vi "Panel.vi"(11 "ButtonControlEditorPanel in":refnum<class "ButtonControlEditorPanel.lvclass">) -> ()   [LabVIEW 2020, in "VolatusGUIControls.lvlib" / "ButtonControlEditorPanel.lvclass"]
uses:
  ButtonControlEditorPanel.lvclass
  C:/dev/lv20CE/relink/volatus-gui-controls/VolatusGUIEditorCore/ElementEditorPanel/ElementEditorPanel.lvclass
  C:/dev/lv20CE/relink/lv-oopanel/OOPanel/Panel/Panel.lvclass
  lv-oopanel/OOPanel/Panel/Basic UI State.ctl
  lv-autocomplete/AutoComplete/AutoComplete/AutoComplete.lvclass/AutoComplete.ctl
  ButtonControlEditorPanel.lvclass/ButtonControlEditorPanel.ctl
  31a50c44-4b6b-485d-bc13-bfcd23764fd1.vi
  03e8aef8-299f-4e90-a8ff-d58387ca9363.vi
  lv-autocomplete/AutoComplete/Launch Autocomplete Handler.vi
  <vilib>/JDP Science/JSONtext/Variant to JSON Text.vi
  <vilib>/JDP Science/JSONtext/Set Item.vi
  <vilib>/JDP Science/JSONtext/Pretty Print.vi
  lv-autocomplete/AutoComplete/AutoComplete/AutoComplete.lvclass
  <vilib>/JDP Science/JSONtext/LVClass Serializer/JSONtext LVClass Serializer.lvclass
  lv-oopanel/OOPanel/Panel/Panel.lvclass
  lv-oopanel/OOPanel/OOPanel.lvlib
  VolatusGUIControls.lvlib
  VolatusGUIEditorCore/ElementEditorPanel/ElementEditorPanel.lvclass
  VolatusGUIEditorCore/VolatusGUIEditorCore.lvlib
panel:
  in  "Inhibit":string caption="Channel"
  in  "Top":i32
  in  "Left":i32
  in  "Height":u16
  in  "Width":u16
  in  "Label Text Color":u32(colorbox) caption="Color"
  in  "Text Color":u32(colorbox)
  in  "Label Visible":bool caption="Visible"
  in  "Label":string
  in  "Multi":bool
  in  "Channel":string
  in  "True Color":u32(colorbox)
  in  "False Color":u32(colorbox)
  in  "True Text":string
  in  "False Text":string
  # "Label"
  # "False"
  # "True"
  # "Text"
  # "BG"
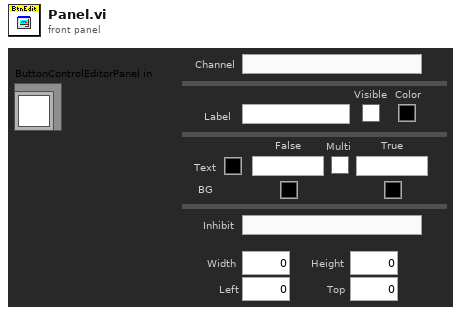
[diagram p1: front panel]
types:
  T1 = typedef "OOPanel.lvlib/Panel.lvclass/Basic UI State.ctl" = enum16{"Init", "Run", "Close"}
  T2 = typedef "VolatusGUIEditorCore.lvlib/ElementEditorPanel.lvclass/Incoming Events.ctl" = cluster{"Update Control":refnum<user-event>}
  T3 = typedef "OOPanel.lvlib/Panel.lvclass/Panel Events.ctl" = cluster{"Visbility":refnum<user-event>, "Close":refnum<user-event>}
  T4 = typedef "VolatusGUIControls.lvlib/ButtonControlEditorPanel.lvclass/Props.ctl" = cluster{"JSON":T5, "Label":T6, "Position":T7, "Width":u16, "Height":u16, "Boolean Colors":T8, "Boolean Text Props":T9}
  T5 = typedef "VolatusGUIControls.lvlib/ButtonControlEditorPanel.lvclass/JSON Props.ctl" = cluster{"Channel":string, "Inhibit":string}
  T6 = typedef "VolatusGUIEditorCore.lvlib/Label Props.ctl" = cluster{"Text":string, "Text Color":u32, "Visible":bool}
  T7 = typedef "VolatusGUIEditorCore.lvlib/Position Props.ctl" = cluster{"Left":i32, "Top":i32}
  T8 = typedef "VolatusGUIEditorCore.lvlib/Boolean Color Props.ctl" = cluster{"False":u32, "True":u32}
  T9 = typedef "VolatusGUIEditorCore.lvlib/Boolean Text Props.ctl" = cluster{"Color":u32, "MultiString":bool, "False":string, "True":string, "Visible":bool}
  T10 = typedef "OOPanel.lvlib/Visibility State.ctl" = enum16{"Idle", "Closed", "Hidden", "Visible", "Subpanel", "Hidden Subpanel"}
  T11 = cluster{"Label":string, "Label Text Color":u32, "Label Visible":bool}
  T12 = cluster{"Text Color":u32, "Multi":bool, "False Text":string, "True Text":string, "Visible":bool}
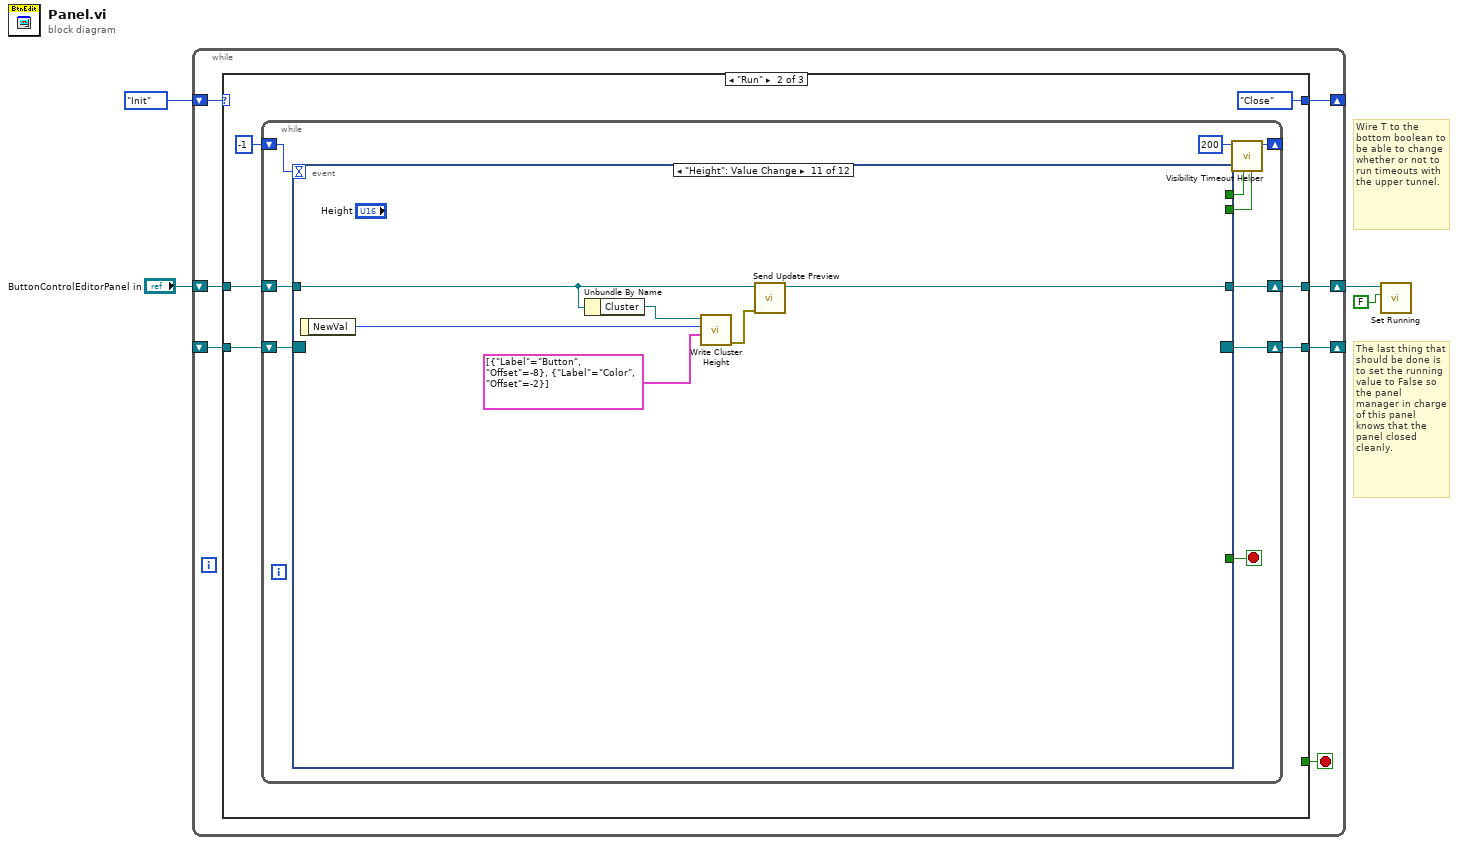
[diagram p0: block diagram]
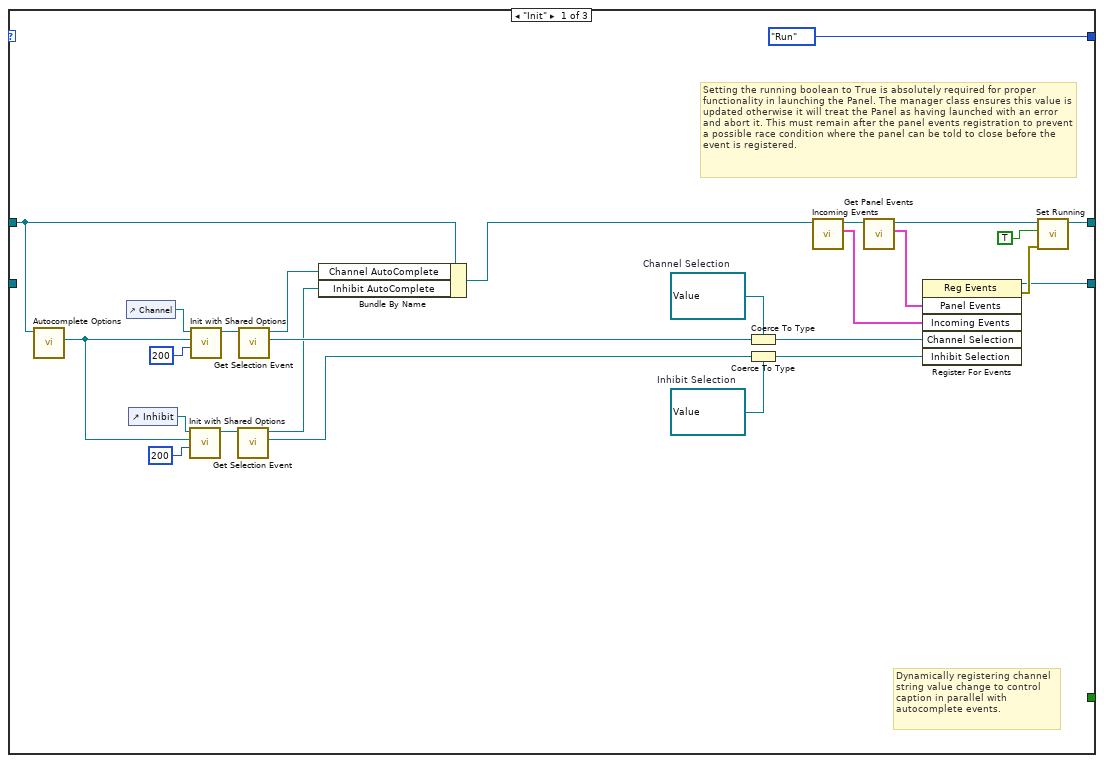
[diagram p2: hidden frame]
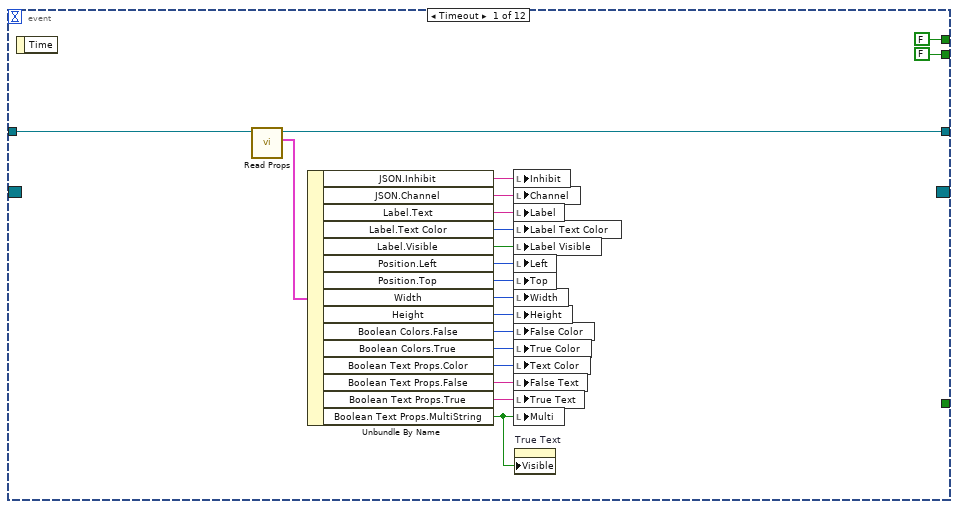
[diagram p3: hidden frame]
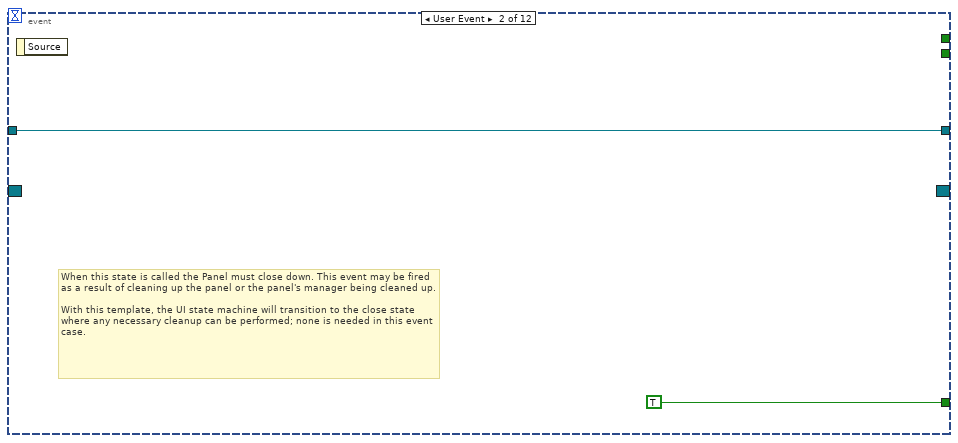
[diagram p4: hidden frame]
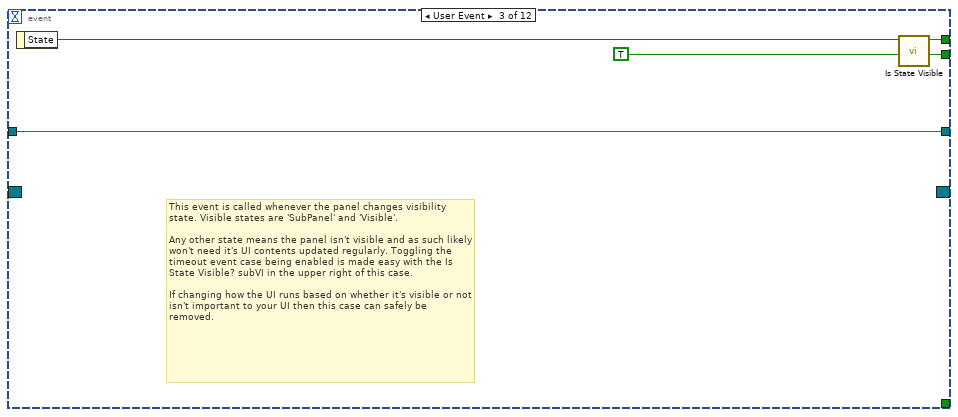
[diagram p5: hidden frame]
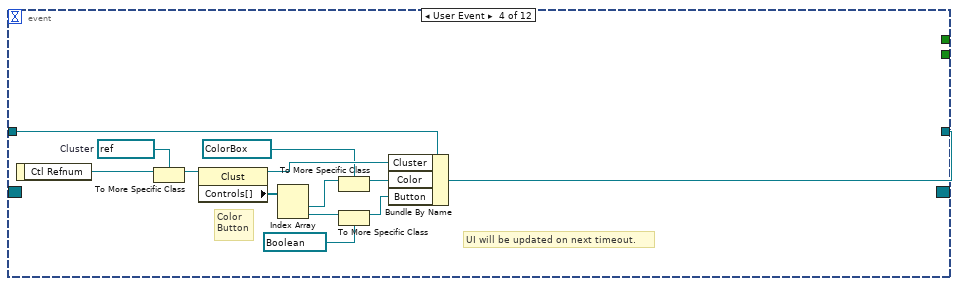
[diagram p6: hidden frame]
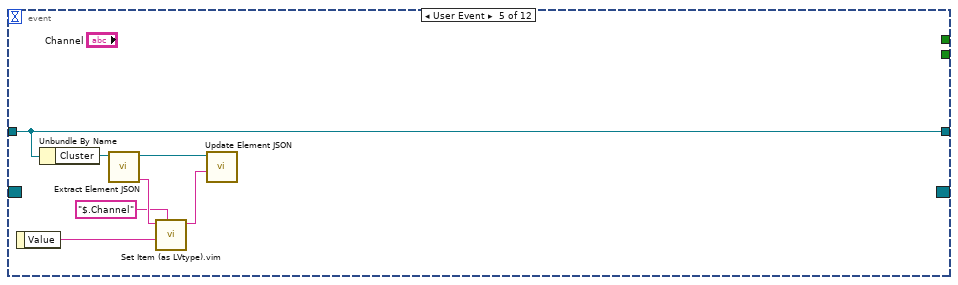
[diagram p7: hidden frame]
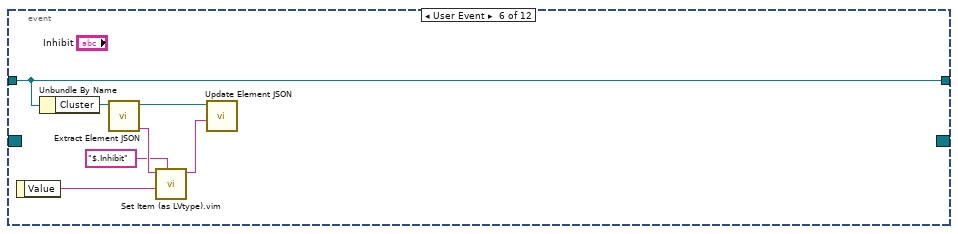
[diagram p8: hidden frame]
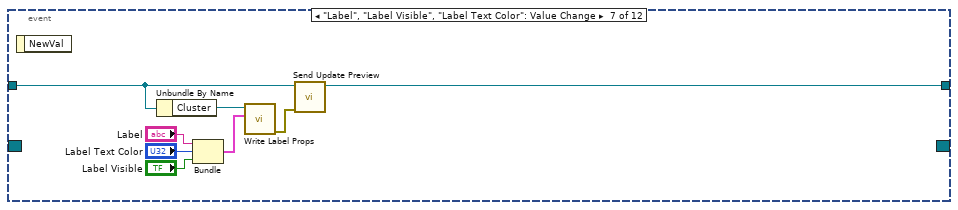
[diagram p9: hidden frame]
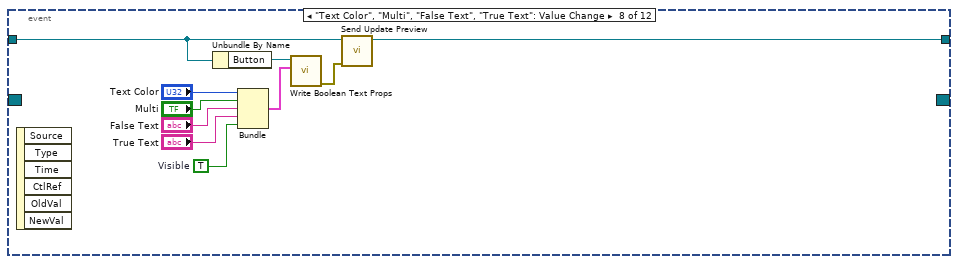
[diagram p10: hidden frame]
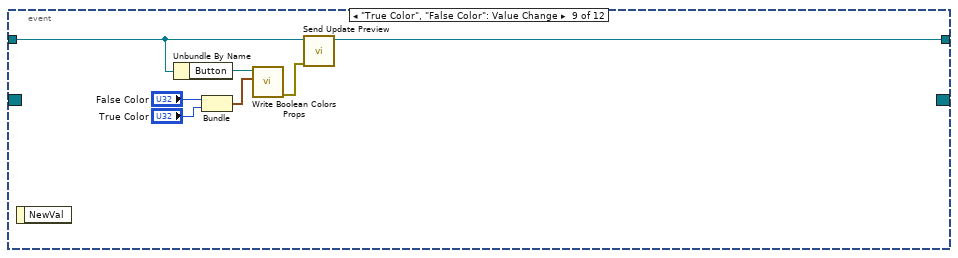
[diagram p11: hidden frame]
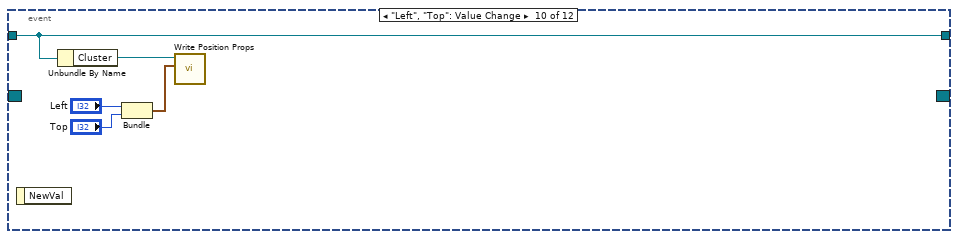
[diagram p12: hidden frame]
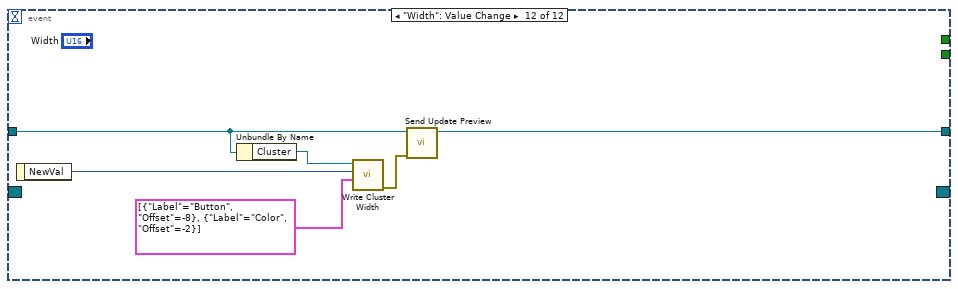
[diagram p13: hidden frame]
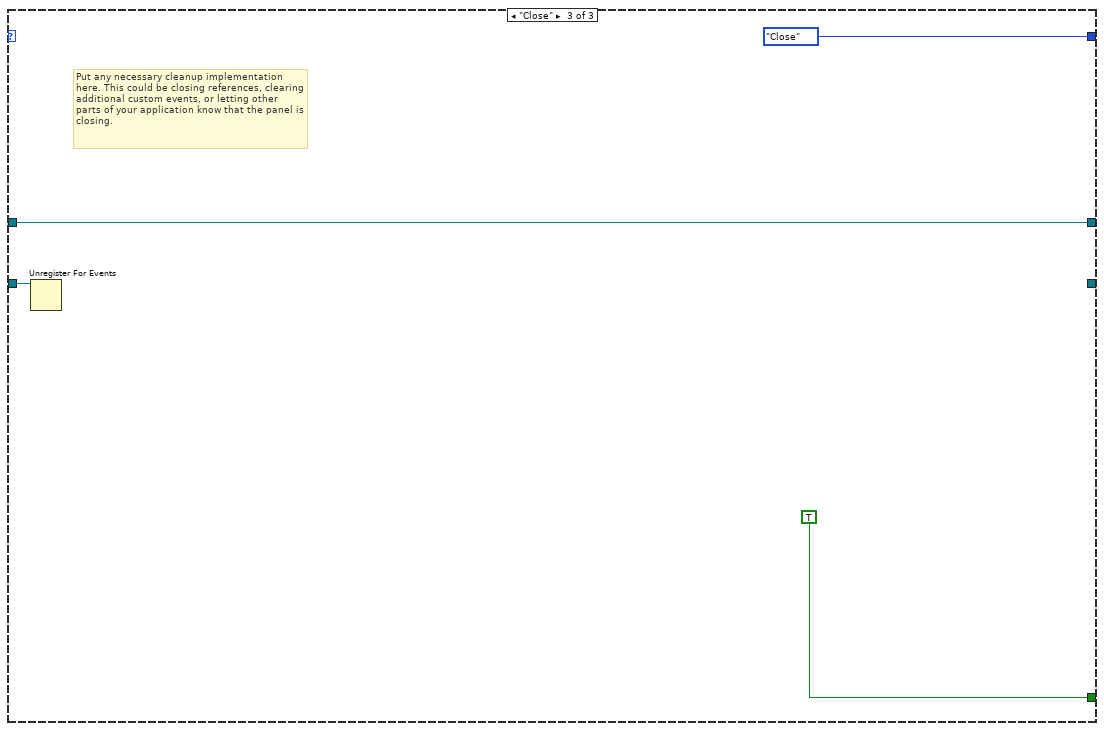
[diagram p14: hidden frame]
diagram:
  # "The last thing that should be done is to set the running value to False so the panel manager in charge of this panel knows that the panel closed cleanly."
  # "Wire T to the bottom boolean to be able to change whether or not to run timeouts with the upper tunnel."
  n1 = while {
    shift-right: [w10] -> _
    shift-left: _ -> [w11]
    shift-right: [w8] -> _
    shift-left: Basic_UI_State."Init" ("Basic UI State") -> [w9]
    shift-right: [w6] -> w4
    shift-left: "ButtonControlEditorPanel in" -> [w5]
    stop <- w7 stop-if-true
    n2 = case shown="\"Run\"" w9 {
      tunnel: w11 -> [_ w43 w150]
      tunnel: [w34 w41 _] -> w10
      tunnel: [Basic_UI_State."Run" ("Basic UI State") Basic_UI_State."Close" ("Basic UI State") Basic_UI_State."Close" ("Basic UI State")] -> w8
      tunnel: [_ _ TRUE] -> w7
      tunnel: [w33 w38 w149] -> w6
      tunnel: w5 -> [w30 w39 w149]
      frame "Init" {
        w12 = refnum<user-event> refnum  # Inhibit Selection
        w14 = refnum<user-event> refnum  # Channel Selection
        # "Dynamically registering channel string value change to control caption in parallel with autocomplete events."
        # "Setting the running boolean to True is absolutely required for proper functionality in launching the Panel. The manager class ensures this value is updated otherwise it will treat the Panel as having launched with an error and abort it. This must remain after the panel events registration to prevent a possible race condition where the panel can be told to close before the event is registered."
        n3 = call "Autocomplete Options.vi"("ElementEditorPanel in"=w30) -> ("Autocomplete Options"=w18:refnum<class "Shared Options.lvclass">)  [unwired: 10 in]
        n4 = control-ref of="Channel"() -> (w29:refnum<vi>)
        n5 = control-ref of="Inhibit"() -> (w19:refnum<vi>)
        n6 = call "Init with Shared Options.vi"("Height (200)"=i16 200, "Shared Options"=w18, "Str Refnum"=w19) -> ("AutoComplete out"=w20:refnum<class "AutoComplete.lvclass">)  [unwired: 7 in, 1 out]
        n7 = call "Init with Shared Options.vi"("Height (200)"=i16 200, "Shared Options"=w18, "Str Refnum"=w29) -> ("AutoComplete out"=w28:refnum<class "AutoComplete.lvclass">)  [unwired: 7 in, 1 out]
        n8 = call "Get Selection Event.vi"("AutoComplete in"=w20) -> ("Selection Event"=w16:refnum<user-event>, "AutoComplete"=w17:refnum<class "AutoComplete.lvclass">)  [unwired: 9 in]
        n9 = call "Get Selection Event.vi"("AutoComplete in"=w28) -> ("Selection Event"=w27:refnum<user-event>, "AutoComplete"=w25:refnum<class "AutoComplete.lvclass">)  [unwired: 9 in]
        n10 = Bundle By Name(cluster=w30, "Channel AutoComplete"=w25, "Inhibit AutoComplete"=w17) -> (w23:refnum<class "ButtonControlEditorPanel.lvclass">)
        n11 = Coerce To Type(0:w27, 1:w14) -> (2:w15:refnum<user-event>)
        n12 = Coerce To Type(0:w16, 1:w12) -> (2:w13:refnum<user-event>)
        n13 = call "Incoming Events.vi"("ElementEditorPanel in"=w23) -> ("Incoming Events"=w24:T2, "ElementEditorPanel out"=w22:refnum<class "ButtonControlEditorPanel.lvclass">)  [unwired: 9 in]
        n14 = call "Get Panel Events.vi"("Panel in"=w22) -> ("Panel Events"=w31:T3, "Panel out"=w32:refnum<class "ButtonControlEditorPanel.lvclass">)  [unwired: 8 in, 1 out]
        n15 = register-events(w31, w24, w15, w13) -> (reference out=w34:refnum<event-registration>, error out=w36:errorcluster)  [unwired: 2 in]
        n16 = call "Set Running.vi"("error in (no error)"=w36, "Running"=TRUE, "Panel in"=w32) -> ("Panel out"=w33:refnum<class "ButtonControlEditorPanel.lvclass">)  [unwired: 7 in, 1 out]
      }
      frame "Run" {
        n17 = while {
          shift-right: [w49] -> w41
          shift-left: w43 -> [w50]
          shift-right: [w52] -> _
          shift-left: -1 ("Timeout") -> [w51]
          shift-right: [w44] -> w38
          shift-left: w39 -> [w45]
          stop <- w46 stop-if-true
          n18 = event shown="[10] \"Height\": Value Change" {
            selector: w50 -> [_ _ _ _ _ _ _ _ _ _ _ _]
            dyn-events: [_ _ _ _ _ _ _ _ _ _ _ _] -> w49
            timeout: w51 -> [_ _ _ _ _ _ _ _ _ _ _ _]
            tunnel: [FALSE _ w78 _ _ _ _ _ _ _ _ _] -> w48
            tunnel: [FALSE _ TRUE _ _ _ _ _ _ _ _ _] -> w47
            tunnel: [_ TRUE _ _ _ _ _ _ _ _ _ _] -> w46
            tunnel: w45 -> [w69 w74 w76 w92 w99 w106 w114 w124 w131 w136 w139 w148]
            tunnel: [w68 w74 w76 w80 w99 w106 w113 w117 w130 w136 w137 w147] -> w44
            event Timeout {
              n19 = event-data() -> ()  [unwired: 1 in, 1 out]
              n20 = call "Read Props.vi"("ButtonControlEditorPanel in"=w69) -> ("Props"=w71:T4, "ButtonControlEditorPanel out"=w68:refnum<class "ButtonControlEditorPanel.lvclass">)  [unwired: 8 in, 1 out]
              n21 = Unbundle By Name(w71) -> ("JSON.Inhibit"=w54:string, "JSON.Channel"=w70:string, "Label.Text"=w67:string, "Label.Text Color"=w65:u32, "Label.Visible"=w64:bool, "Position.Left"=w63:i32, "Position.Top"=w62:i32, "Width"=w61:u16, "Height"=w60:u16, "Boolean Colors.False"=w59:u32, "Boolean Colors.True"=w58:u32, "Boolean Text Props.Color"=w57:u32, "Boolean Text Props.False"=w56:string, "Boolean Text Props.True"=w66:string, "Boolean Text Props.MultiString"=w55:bool)
              n22 = local write "Inhibit"(w54) -> ()
              n23 = local write "Channel"(w70) -> ()
              n24 = local write "Label"(w67) -> ()
              n25 = local write "Label Text Color"(w65) -> ()
              n26 = local write "Label Visible"(w64) -> ()
              n27 = local write "Left"(w63) -> ()
              n28 = local write "Top"(w62) -> ()
              n29 = local write "Width"(w61) -> ()
              n30 = local write "Height"(w60) -> ()
              n31 = local write "False Color"(w59) -> ()
              n32 = local write "True Color"(w58) -> ()
              n33 = local write "Text Color"(w57) -> ()
              n34 = local write "False Text"(w56) -> ()
              n35 = local write "True Text"(w66) -> ()
              n36 = local write "Multi"(w55) -> ()
              n37 = property on="True Text" class="Str"("Visible"=w55) -> ()  [unwired: 2 in, 2 out]
            }
            event User Event {
              # "When this state is called the Panel must close down. This event may be fired as a result of cleaning up the panel or the panel's manager being cleaned up.\n\nWith this template, the UI state machine will transition to the close state where any necessary cleanup can be performed; none is needed in this event case."
              n38 = event-data() -> ()  [unwired: 1 in, 1 out]
            }
            event User Event {
              # "This event is called whenever the panel changes visibility state. Visible states are 'SubPanel' and 'Visible'.\n\nAny other state means the panel isn't visible and as such likely won't need it's UI contents updated regularly. Toggling the timeout event case being enabled is made easy with the Is State Visible? subVI in the upper right of this case.\n\nIf changing how the UI runs based on whether it's visible or not isn't important to your UI then this case can safely be removed."
              n39 = event-data() -> ("State"=w79:T10)  [unwired: 1 in]
              n40 = call "Is State Visible.vi"("Visibility"=w79) -> ("Visible"=w78:bool)  [unwired: 10 in]
            }
            event User Event {
              w89 = refnum<vi> refnum  # Cluster
              # "UI will be updated on next timeout."
              # "Color\nButton"
              n41 = event-data() -> ("Ctl Refnum"=w91:refnum<vi>)  [unwired: 1 in]
              n42 = To More Specific Class(target class=w89, reference=w91) -> (specific class reference=w90:refnum<vi>)  [unwired: 1 in, 1 out]
              n43 = property class="Clust"(reference=w90) -> (reference out=w85:refnum<vi>, "Controls[]"=w88:refnum<vi>[])  [unwired: 1 in, 1 out]
              n44 = Index Array(array=w88) -> (element #1=w82:refnum<vi>, element #2=w87:refnum<vi>)  [unwired: 2 in]
              n45 = To More Specific Class(target class=refnum<vi> refnum ("False Color"), reference=w82) -> (specific class reference=w83:refnum<vi>)  [unwired: 1 in, 1 out]
              n46 = To More Specific Class(target class=refnum<vi> refnum ("Button"), reference=w87) -> (specific class reference=w84:refnum<vi>)  [unwired: 1 in, 1 out]
              n47 = Bundle By Name(cluster=w92, "Cluster"=w85, "Color"=w83, "Button"=w84) -> (w80:refnum<class "ButtonControlEditorPanel.lvclass">)
            }
            event User Event {
              n48 = event-data() -> ("Value"=w96:string)  [unwired: 1 in]
              n49 = Unbundle By Name(w99) -> ("Cluster"=w98:refnum<vi>)
              n50 = call "Extract Element JSON.vi"("Ctl Refnum in"=w98) -> ("JSON"=w97:string, "Ctl Refnum"=w94:refnum<vi>)  [unwired: 7 in, 2 out]
              n51 = call "Set Item (as LVtype).vim"("$Path or Item Name"="$.Channel", "Anything"=w96, "JSON"=w97) -> ("<JSON>"=w93:string)  [unwired: 5 in, 2 out]
              n52 = call "Update Element JSON.vi"("JSON"=w93, "Ctl Refnum in"=w94) -> ()  [unwired: 8 in, 2 out]
            }
            event User Event {
              n53 = event-data() -> ("Value"=w103:string)  [unwired: 1 in]
              n54 = Unbundle By Name(w106) -> ("Cluster"=w105:refnum<vi>)
              n55 = call "Extract Element JSON.vi"("Ctl Refnum in"=w105) -> ("JSON"=w104:string, "Ctl Refnum"=w101:refnum<vi>)  [unwired: 7 in, 2 out]
              n56 = call "Set Item (as LVtype).vim"("$Path or Item Name"="$.Inhibit", "Anything"=w103, "JSON"=w104) -> ("<JSON>"=w100:string)  [unwired: 5 in, 2 out]
              n57 = call "Update Element JSON.vi"("JSON"=w100, "Ctl Refnum in"=w101) -> ()  [unwired: 8 in, 2 out]
            }
            event "Label", "Label Visible", "Label Text Color": Value Change {
              n58 = event-data() -> ()  [unwired: 1 in, 1 out]
              n59 = Unbundle By Name(w114) -> ("Cluster"=w112:refnum<vi>)
              n60 = Bundle("Label"="Label", "Label Text Color"="Label Text Color", "Label Visible"="Label Visible") -> (w107:T11)  [unwired: 1 in]
              n61 = call "Write Label Props.vi"("Label Props"=w107, "Ctl Refnum in"=w112) -> ("error out"=w111:errorcluster)  [unwired: 8 in, 1 out]
              n62 = call "Send Update Preview.vi"("error in (no error)"=w111, "ElementEditorPanel in"=w114) -> ("ElementEditorPanel out"=w113:refnum<class "ButtonControlEditorPanel.lvclass">)  [unwired: 8 in, 1 out]
            }
            event "Text Color", "Multi", "False Text", "True Text": Value Change {
              w115 = TRUE  # Visible
              n63 = event-data() -> ()  [unwired: 1 in, 6 out]
              n64 = Unbundle By Name(w124) -> ("Button"=w119:refnum<vi>)
              n65 = Bundle("Text Color"="Text Color", "Multi"="Multi", "False Text"="False Text", "True Text"="True Text", "Visible"=w115) -> (w118:T12)  [unwired: 1 in]
              n66 = call "Write Boolean Text Props.vi"("Boolean Text Props"=w118, "Control In"=w119) -> ("error out"=w116:errorcluster)  [unwired: 8 in, 1 out]
              n67 = call "Send Update Preview.vi"("error in (no error)"=w116, "ElementEditorPanel in"=w124) -> ("ElementEditorPanel out"=w117:refnum<class "ButtonControlEditorPanel.lvclass">)  [unwired: 8 in, 1 out]
            }
            event "True Color", "False Color": Value Change {
              n68 = event-data() -> ()  [unwired: 1 in, 1 out]
              n69 = Unbundle By Name(w131) -> ("Button"=w129:refnum<vi>)
              n70 = Bundle("False Color"="False Color", "True Color"="True Color") -> (w126:cluster{"False Color":u32, "True Color":u32})  [unwired: 1 in]
              n71 = call "Write Boolean Colors Props.vi"("Boolean Colors Props"=w126, "Control in"=w129) -> ("error out"=w125:errorcluster)  [unwired: 8 in, 1 out]
              n72 = call "Send Update Preview.vi"("error in (no error)"=w125, "ElementEditorPanel in"=w131) -> ("ElementEditorPanel out"=w130:refnum<class "ButtonControlEditorPanel.lvclass">)  [unwired: 8 in, 1 out]
            }
            event "Left", "Top": Value Change {
              n73 = event-data() -> ()  [unwired: 1 in, 1 out]
              n74 = Unbundle By Name(w136) -> ("Cluster"=w135:refnum<vi>)
              n75 = Bundle("Left"="Left", "Top"="Top") -> (w132:cluster{"Left":i32, "Top":i32})  [unwired: 1 in]
              n76 = call "Write Position Props.vi"("Position Props"=w132, "Ctl Refnum in"=w135) -> ()  [unwired: 8 in, 2 out]
            }
            event "Height": Value Change {
              n77 = event-data() -> ("NewVal"=w138:u16)  [unwired: 1 in]
              n78 = Unbundle By Name(w139) -> ("Cluster"=w142:refnum<vi>)
              n79 = call "Write Cluster Height.vi"("Nested Offsets (None)"=cluster{"Label":string, "Offset":i32}[] [{"Label"="Button", "Offset"=-8}, {"Label"="Color", "Offset"=-2}], "Height"=w138, "Cluster in"=w142) -> ("error out"=w140:errorcluster)  [unwired: 7 in, 1 out]
              n80 = call "Send Update Preview.vi"("error in (no error)"=w140, "ElementEditorPanel in"=w139) -> ("ElementEditorPanel out"=w137:refnum<class "ButtonControlEditorPanel.lvclass">)  [unwired: 8 in, 1 out]
            }
            event "Width": Value Change {
              n81 = event-data() -> ("NewVal"=w145:u16)  [unwired: 1 in]
              n82 = Unbundle By Name(w148) -> ("Cluster"=w146:refnum<vi>)
              n83 = call "Write Cluster Width.vi"("Nested Offsets (None)"=cluster{"Label":string, "Offset":i32}[] [{"Label"="Button", "Offset"=-8}, {"Label"="Color", "Offset"=-2}], "Width"=w145, "Cluster in"=w146) -> ("error out"=w143:errorcluster)  [unwired: 7 in, 1 out]
              n84 = call "Send Update Preview.vi"("error in (no error)"=w143, "ElementEditorPanel in"=w148) -> ("ElementEditorPanel out"=w147:refnum<class "ButtonControlEditorPanel.lvclass">)  [unwired: 8 in, 1 out]
            }
          }
          n85 = call "Visibility Timeout Helper.vi"("Update?"=w47, "Use Timeout?"=w48, "Visible Timeout mS"=200) -> ("Timeout"=w52:i32)  [unwired: 8 in]
        }
      }
      frame "Close" {
        # "Put any necessary cleanup implementation here. This could be closing references, clearing additional custom events, or letting other parts of your application know that the panel is closing."
        n86 = Unregister For Events(event registration refnum=w150) -> ()  [unwired: 1 in, 1 out]
      }
    }
  }
  n87 = call "Set Running.vi"("Running"=FALSE, "Panel in"=w4) -> ()  [unwired: 8 in, 2 out]
